vi "DesignForm.vi"(11 "httpRequestID":u32) -> ()   [LabVIEW 2011, in "Design Server.lvlib"]
uses:
  AguaClara Design Server/Design Server.lvlib
  ADT 2/user project design.ctl
  <vilib>/wsapi/NI_WebServices.lvlib
panel:
  out "Design exists":bool
  in  "error in (no error)":errorcluster
  out "request variables":T1
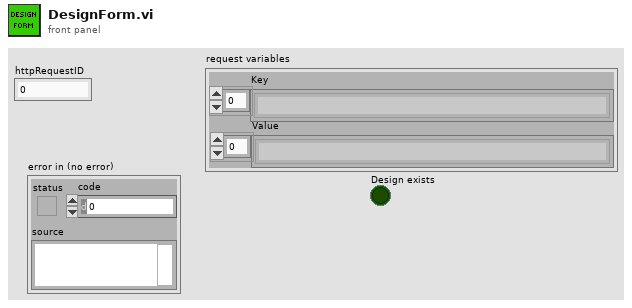
[diagram p1: front panel]
types:
  T1 = typedef "user project design.ctl" = cluster{"Key":string[], "Value":string[]}
  T2 = typedef "Design Server.lvlib/Design Request.ctl" = cluster{"Project Folder":path, "Method Name":string, "Inputs":T3, "Version":i32}
  T3 = typedef "Design Server.lvlib/Variable cluster.ctl" = cluster{"Label.Text":string, "Control Type":u32, "Numeric":dbl, "Array":dbl[], "status":bool, "Str Array":string[], "String":string, "unit":string}[]
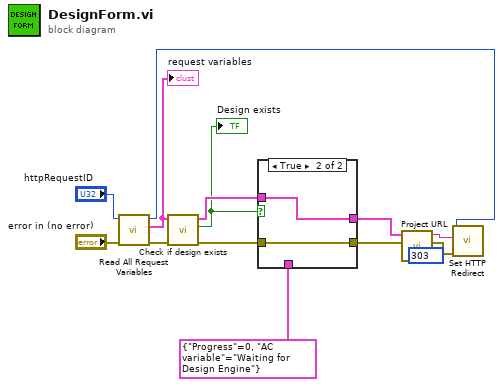
[diagram p0: block diagram]
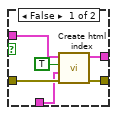
[diagram p2: hidden frame]
diagram:
  w1 = 303 items=["100"=100, "101"=101, "200"=200, "201"=201, "202"=202, "203"=203, "204"=204, "205"=205, "206"=206, "300"=300, "301"=301, "302"=302, "303"=303, "304"=304, "305"=305, "306"=306, "307"=307, "400"=400, "401"=401, "402"=402, "403"=403, "404"=404, "405"=405, "406"=406, "407"=407, "408"=408, "409"=409, "410"=410, "411"=411, "412"=412, "413"=413, "414"=414, "415"=415, "416"=416, "417"=417, "500"=500, "501"=501, "502"=502, "503"=503, "504"=504, "505"=505] ("response code (307)")
  n1 = call <vilib>:"Read All Request Variables.vi"("error in (no error)"="error in (no error)", "httpRequestID"="httpRequestID") -> ("error out"=w11:errorcluster, "request variables"=w10:cluster{"Key":string[], "Value":string[]}, "httpRequestID out"=w3:u32)  [unwired: 7 in]
  "request variables" <- w10
  n2 = call "Check if design exists.vi"("error in"=w11, "Request"=w10) -> ("error out"=w7:errorcluster, "Design exists"=w6:bool, "DesignRequest"=w8:T2)  [unwired: 5 in, 2 out]
  "Design exists" <- w6
  n3 = case shown="True" w6 {
    tunnel: [w17 w22] -> w13
    tunnel: [w18 w21] -> w9
    tunnel: w8 -> [w20 w22]
    tunnel: w7 -> [w19 w21]
    tunnel: cluster{"Progress":u8, "AC variable":string} {"Progress"=0, "AC variable"="Waiting for Design Engine"} ("progress") -> [w16 _]
    frame False {
      n4 = call "Create html index.vi"("error in"=w19, "progress"=w16, "Under construction"=TRUE, "DesignRequest"=w20) -> ("error out"=w18:errorcluster, "DesignRequest out"=w17:T2)  [unwired: 6 in]
    }
    frame True {
    }
  }
  n5 = call "Project URL.vi"("error in (no error)"=w9, "DesignRequest"=w13) -> ("error out"=w2:errorcluster, "Project URL"=w4:string)  [unwired: 8 in]
  n6 = call <vilib>:"Set HTTP Redirect.vi"("error in (no error)"=w2, "response code (307)"=w1, "redirect URL"=w4, "httpRequestID"=w3) -> ()  [unwired: 6 in, 2 out]
